vi "HSOpMuxNoRef.vi"() -> ()   [LabVIEW 2013]
uses:
  Multiplexer_Opmux.lvclass
  OverallRoutines/HS3OverallRoutines.lvlib
panel:
  out "tmr":u32 caption="Elapsed for acq"
  in  "Run":bool
  out "Ch8":dbl[](graph)
  out "Ch7":dbl[](graph)
  out "Ch6":dbl[](graph)
  out "Ch5":dbl[](graph)
  out "Ch4":dbl[](graph)
  out "Ch3":dbl[](graph)
  out "Ch2":dbl[](graph)
  out "Ch1":dbl[](graph)
  in  "Scan":bool
  in  "Set":bool
  in  "Length":dbl=1.0 caption="Length (us)" min=0.1 max=6.3 step=0.1
  in  "Voltage":dbl min=0.0 max=1023.0 step=1.0
  in  "Into":u16[](array[numeric])
  in  "Forward":u16[](array[numeric])
  in  "Signal Frequency":u32(ring)=10000000 items=["5Mhz"=5000000, "10Mhz"=10000000, "25Mhz"=25000000]
  in  "Shutdown":bool
  out "Acq":bool caption="Acquiring"
  out "SampleFrequency":dbl format="%#_8g"
  out "ChArray":dbl[](array[numeric])
  out "Serial":i32
  out "DllPath":path
  out "HandyScope":bool
  out "Multiplexer":bool
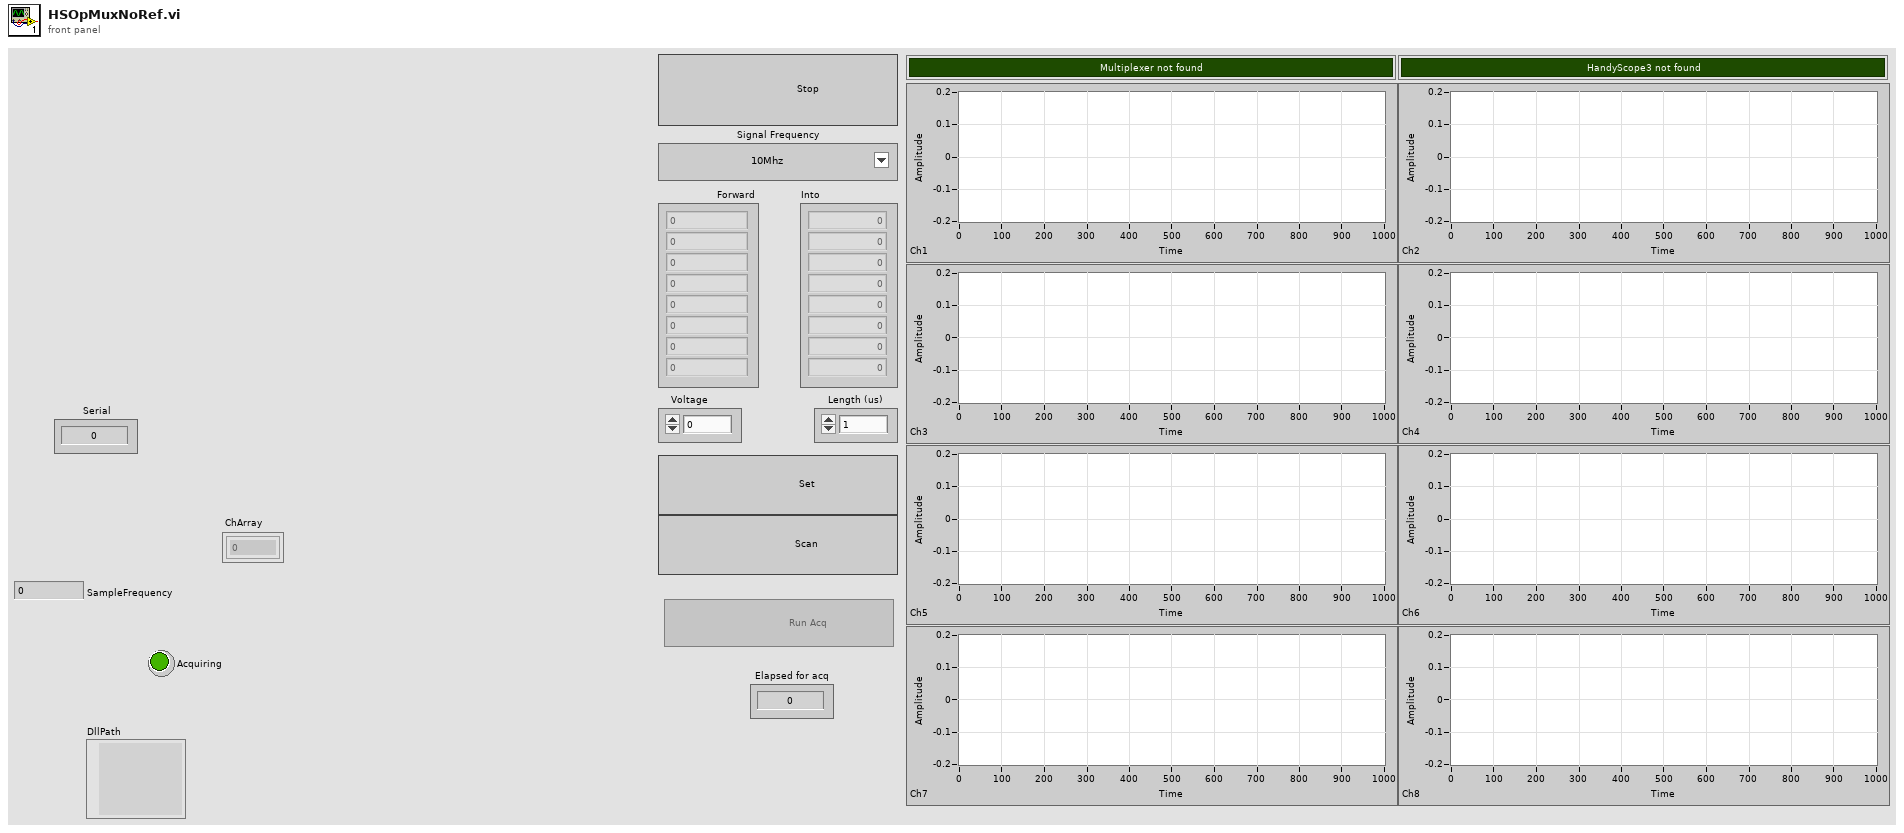
[diagram p1: front panel]
types:
  T1 = cluster{"trgSource":u16, "trgMode":u16, "trgLevel":dbl}
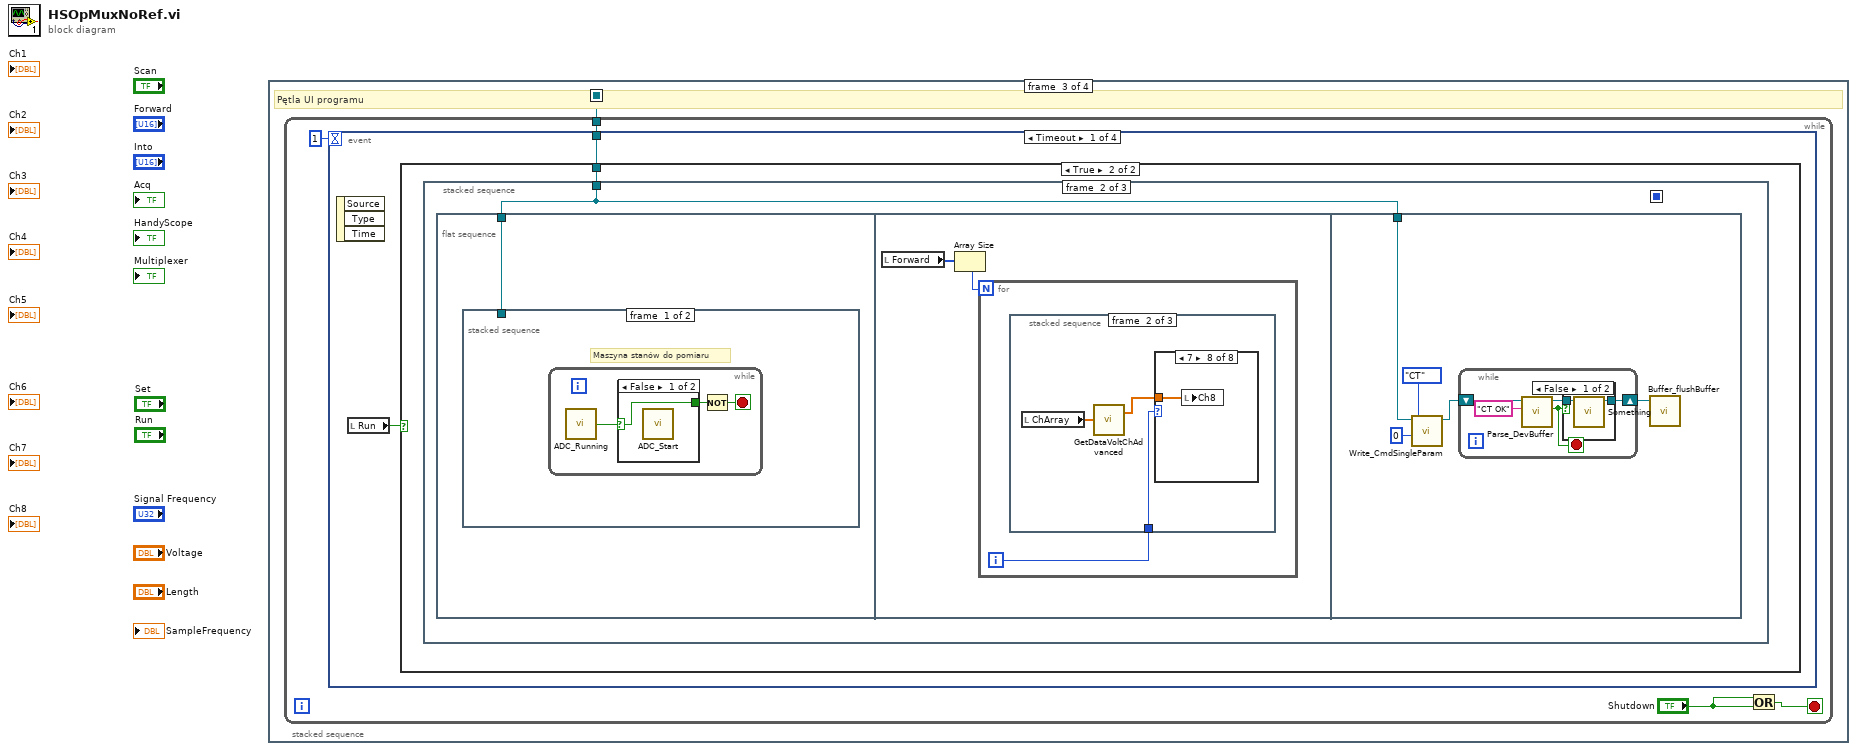
[diagram p0: block diagram]
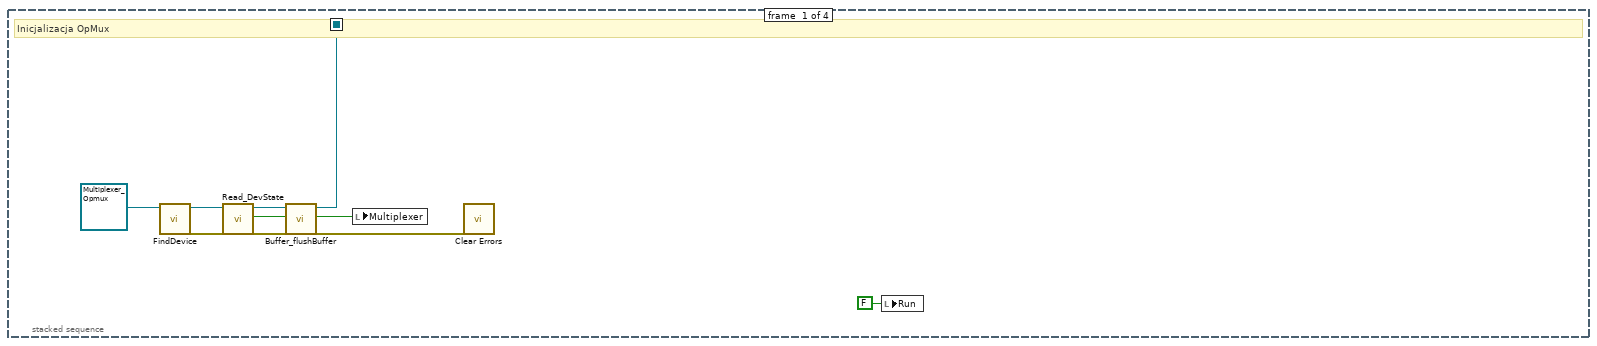
[diagram p2: hidden frame]
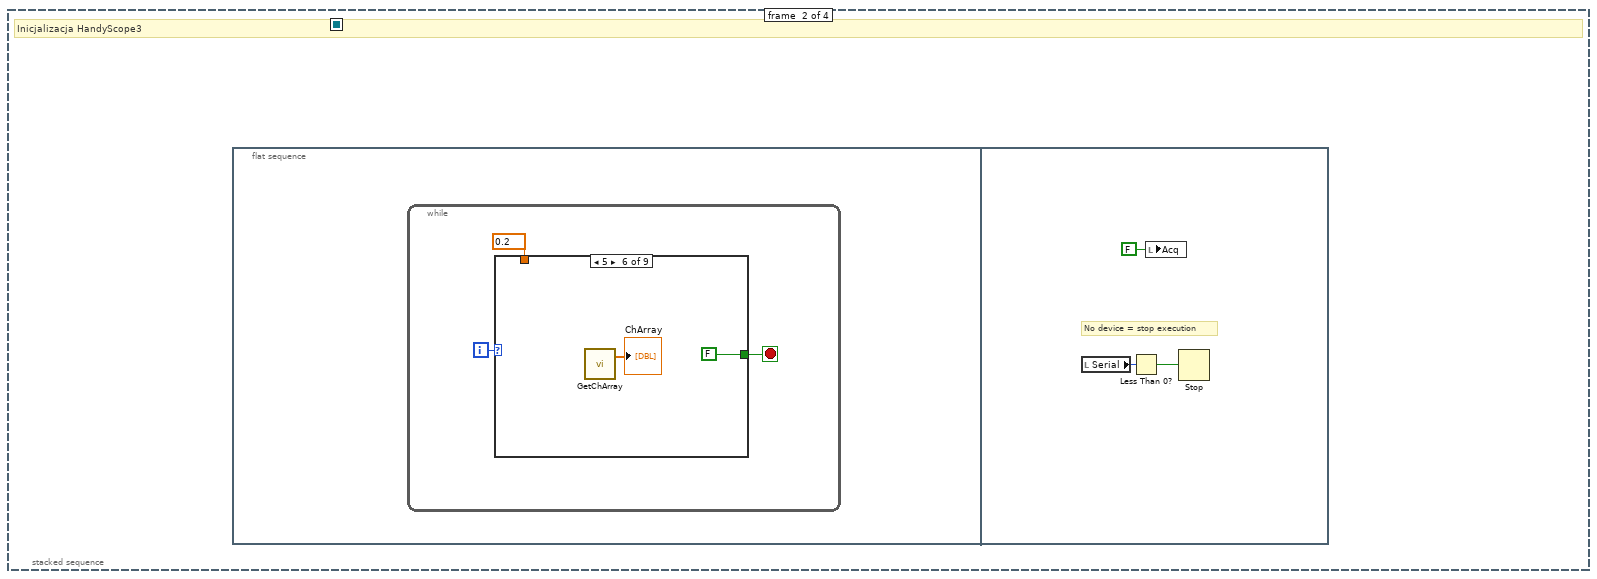
[diagram p3: hidden frame]
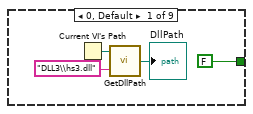
[diagram p4: hidden frame]
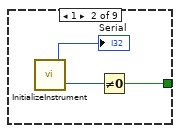
[diagram p5: hidden frame]
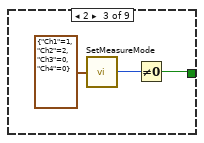
[diagram p6: hidden frame]
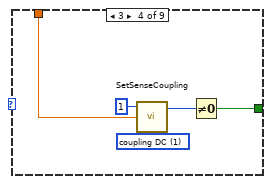
[diagram p7: hidden frame]
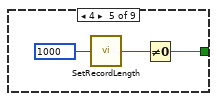
[diagram p8: hidden frame]
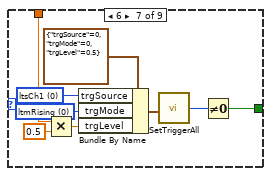
[diagram p9: hidden frame]
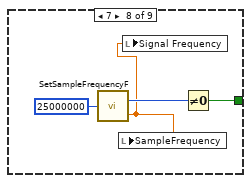
[diagram p10: hidden frame]
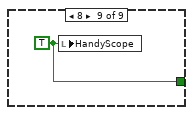
[diagram p11: hidden frame]
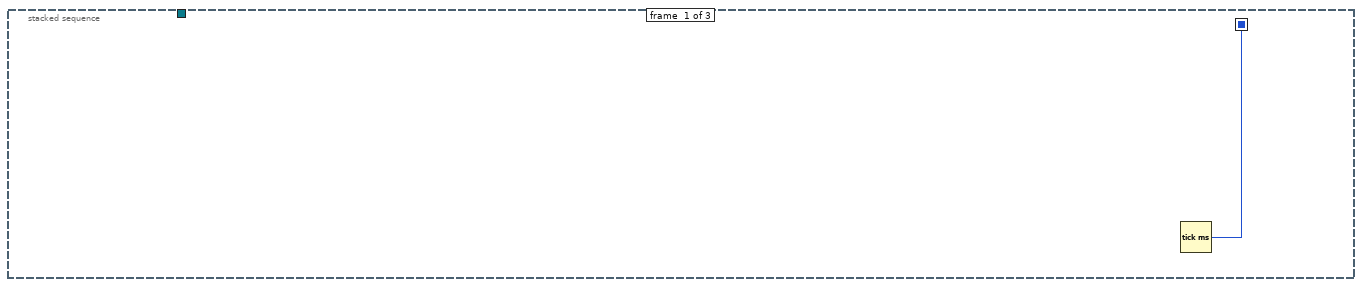
[diagram p13: hidden frame]
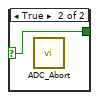
[diagram p14: hidden frame]
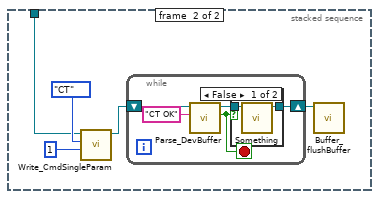
[diagram p15: hidden frame]
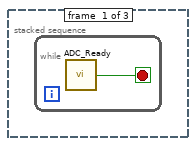
[diagram p17: hidden frame]
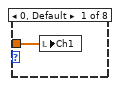
[diagram p18: hidden frame]
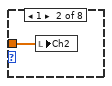
[diagram p19: hidden frame]
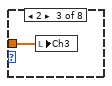
[diagram p20: hidden frame]
diagram:
  n1 = stacked-sequence {
    seq-local: [w1 _ _ _] -> [_ _ w50 _]
    frame #0 {
      # "Inicjalizacja OpMux"
      n2 = call-dynamic "FindDevice.vi"("Multiplexer_Opmux in"=refnum<class "Multiplexer_Opmux.lvclass"> refnum) -> ("error out"=w6:errorcluster, "Multiplexer_Opmux out"=w8:refnum<class "Multiplexer_Opmux.lvclass">)  [unwired: 8 in, 1 out]
      n3 = call-dynamic "Read_DevState.vi"("error in (no error)"=w6, "Multiplexer_Opmux in"=w8) -> ("error out"=w3:errorcluster, "DevState"=w7:bool, "Multiplexer_Opmux out"=w4:refnum<class "Multiplexer_Opmux.lvclass">)  [unwired: 7 in]
      n4 = call-dynamic "Buffer_flushBuffer.vi"("error in (no error)"=w3, "Multiplexer_Opmux in"=w4) -> ("error out"=w2:errorcluster, "Multiplexer_Opmux out"=w1:refnum<class "Multiplexer_Opmux.lvclass">)  [unwired: 8 in]
      n5 = local write "Multiplexer"(w7) -> ()
      n6 = call <vilib>:"Clear Errors.vi"("error in (no error)"=w2) -> ()  [unwired: 6 in, 1 out]
      n7 = local write "Run"(FALSE ("Run")) -> ()
    }
    frame #1 {
      # "Inicjalizacja HandyScope3"
      n8 = flat-sequence {
        frame #0 {
          n9 = while {
            i -> [w12]
            stop <- w11 stop-if-true
            w10 = 0.2 items=["0,2"=0.2, "0,8"=0.8, "2"=2.0, "4"=4.0, "20"=20.0, "40"=40.0, "80"=80.0] ("chSense")
            n10 = case shown="5" w12 {
              tunnel: [FALSE w17 w21 w24 w29 FALSE w40 w45 w46] -> w11
              tunnel: w10 -> [_ _ _ w23 _ _ w36 _ _]
              frame 0, Default {
                n11 = Current VI's Path() -> (path=w14:path)
                n12 = call "GetDllPath.vi"("DllName"="DLL3\\hs3.dll", "path"=w14) -> ("DllPath"=→"DllPath":path)
              }
              frame 1 {
                n13 = call "InitializeInstrument.vi"() -> ("ErrorCode"=w18:i16, "Serial"=→"Serial":i32)
                n14 = Not Equal To 0?(x=w18) -> (x != 0?=w17:bool)
              }
              frame 2 {
                n15 = call "SetMeasureMode.vi"("oModeStack"=cluster{"Ch1":u8, "Ch2":u8, "Ch3":u8, "Ch4":u8} {"Ch1"=1, "Ch2"=2, "Ch3"=0, "Ch4"=0}) -> ("ErrorCode"=w20:i16)
                n16 = Not Equal To 0?(x=w20) -> (x != 0?=w21:bool)
              }
              frame 3 {
                w27 = 1 items=["coupling AC", "coupling DC"] ("chCoupling")
                n17 = call "SetSenseCoupling.vi"("chCoupling"=w27, "chSense"=w23, "chSet"=1) -> ("ErrorCode"=w25:i16)  [unwired: 1 out]
                n18 = Not Equal To 0?(x=w25) -> (x != 0?=w24:bool)
              }
              frame 4 {
                w30 = u32 1000 items=["100"=100, "250"=250, "500"=500, "1000"=1000, "2500"=2500, "5000"=5000, "10000"=10000, "25000"=25000, "50000"=50000, "100000"=100000, "131000"=131000] ("RecordLength")
                n19 = call "SetRecordLength.vi"("RecordLength"=w30) -> ("ErrorCode"=w28:i16)
                n20 = Not Equal To 0?(x=w28) -> (x != 0?=w29:bool)
              }
              frame 5 {
                n21 = call "GetChArray.vi"() -> ("ChArray"=→"ChArray":dbl[])  [unwired: 1 out]
              }
              frame 6 {
                w33 = u16 0 items=["ltmRising", "ltmFalling", "ltmInWindow", "ltmOutWindow", "ltmTVLine", "ltmTVFieldOdd", "ltmTVFieldEven"] ("trgMode")
                w34 = u16 0 items=["ltsCh1"=0, "ltsCh2"=1, "ltsExternal"=4, "ltsAnalogExt"=5, "ltsAnd"=6, "ltsOr"=7, "ltsXor"=8, "ltsNoTrig"=9, "notUsed"=10, "ltsPxiExt"=11, "ltsGenStart"=12, "ltsGenStop"=13, "ltsGenNew"=14] ("trgSource")
                n22 = Multiply(x=w36, y=0.5) -> (x*y=w37:dbl)
                n23 = Bundle By Name(cluster=T1 {"trgSource"=0, "trgMode"=0, "trgLevel"=0.5} ("TriggerSettings"), "trgSource"=w34, "trgMode"=w33, "trgLevel"=w37) -> (w38:T1)
                n24 = call "SetTriggerAll.vi"("TriggerSettings"=w38) -> ("ErrorCode"=w41:i32)
                n25 = Not Equal To 0?(x=w41) -> (x != 0?=w40:bool)
              }
              frame 7 {
                n26 = call "SetSampleFrequencyF.vi"("Numeric Control"=u32 25000000) -> ("ErrorCode"=w44:i16, "oFreq_Set"=w43:dbl)
                n27 = local write "SampleFrequency"(w43) -> ()
                n28 = local write "Signal Frequency"(w43) -> ()
                n29 = Not Equal To 0?(x=w44) -> (x != 0?=w45:bool)
              }
              frame 8 {
                w46 = TRUE ("HandyScope")
                n30 = local write "HandyScope"(w46) -> ()
              }
            }
          }
        }
        frame #1 {
          # "No device = stop execution"
          n31 = local read "Serial"() -> (w49:i32)
          n32 = Less Than 0?(x=w49) -> (x < 0?=w48:bool)
          n33 = local write "Acq"(FALSE ("Acq")) -> ()
          n34 = Stop(stop? (T)=w48) -> ()
        }
      }
    }
    frame #2 {
      # "Pętla UI programu"
      n35 = while {
        tunnel: w50 -> [w51]
        stop <- w53 stop-if-true
        n36 = event shown="[0] Timeout" {
          selector: _ -> [_ _ _ _]
          dyn-events: _ -> [_ _ _ _]
          timeout: 1 -> [_ _ _ _]
          tunnel: w51 -> [w56 _ w111 _]
          event Timeout {
            n37 = event-data() -> ()  [unwired: 1 in, 3 out]
            n38 = local read "Run"() -> (w55:bool)
            n39 = case shown="True" w55 {
              tunnel: w56 -> [_ w57]
              frame False {
              }
              frame True {
                n40 = stacked-sequence {
                  seq-local: [w58 _ _] -> [_ _ w108]
                  tunnel: w57 -> [_ w59 _]
                  frame #0 {
                    n41 = Tick Count (ms)() -> (millisecond timer value=w58:u32)
                  }
                  frame #1 {
                    n42 = flat-sequence {
                      tunnel: w59 -> [w60]
                      tunnel: w59 -> [w96]
                      frame #0 {
                        n43 = stacked-sequence {
                          tunnel: w60 -> [_ w66]
                          frame #0 {
                            # "Maszyna stanów do pomiaru"
                            n44 = while {
                              stop <- w62 stop-if-true
                              n45 = call "ADC_Running.vi"() -> ("Measuring"=w63:bool)
                              n46 = case shown="False" w63 {
                                selector: w63 -> [w64 w65]
                                tunnel: [w64 w65] -> w61
                                frame False {
                                n47 = call "ADC_Start.vi"() -> ()  [unwired: 1 out]
                                }
                                frame True {
                                n48 = call "ADC_Abort.vi"() -> ()  [unwired: 1 out]
                                }
                              }
                              n49 = Not(x=w61) -> (.not. x?=w62:bool)
                            }
                          }
                          frame #1 {
                            n50 = call-dynamic "Write_CmdSingleParam.vi"("Param"=1, "Command"=enum16{"SA", "GT", "SI", "SL", "ST", "CT"}."CT", "Multiplexer_Opmux in"=w66) -> ("Multiplexer_Opmux out"=w68:refnum<class "Multiplexer_Opmux.lvclass">)  [unwired: 7 in, 1 out]
                            n51 = while {
                              shift-right: [w72] -> w67
                              shift-left: w68 -> [w71]
                              stop <- w74 stop-if-true
                              n52 = call-dynamic "Parse_DevBuffer.vi"("searchFor"="CT OK", "Multiplexer_Opmux in"=w71) -> ("Found"=w74:bool, "Multiplexer_Opmux out"=w75:refnum<class "Multiplexer_Opmux.lvclass">)  [unwired: 7 in, 1 out]
                              n53 = case shown="False" w74 {
                                tunnel: w75 -> [w77 w78]
                                tunnel: [w76 w78] -> w72
                                frame False {
                                n54 = call-dynamic "Something.vi"("Multiplexer_Opmux in"=w77) -> ("Multiplexer_Opmux out"=w76:refnum<class "Multiplexer_Opmux.lvclass">)  [unwired: 9 in, 1 out]
                                }
                                frame True {
                                }
                              }
                            }
                            n55 = call-dynamic "Buffer_flushBuffer.vi"("Multiplexer_Opmux in"=w67) -> ()  [unwired: 9 in, 2 out]
                          }
                        }
                      }
                      frame #1 {
                        n56 = local read "Forward"() -> (w80:u16[])
                        n57 = Array Size(array=w80) -> (size(s)=w79:i32)
                        n58 = for {
                          N: w79 -> [_]
                          i -> [w81]
                          n59 = stacked-sequence {
                            tunnel: w81 -> [_ w85 _]
                            frame #0 {
                              n60 = while {
                                stop <- w82 stop-if-true
                                n61 = call "ADC_Ready.vi"() -> ("Ready"=w82:bool)
                              }
                            }
                            frame #1 {
                              n62 = local read "ChArray"() -> (w83:dbl[])
                              n63 = call "GetDataVoltChAdvanced.vi"("chData"=w83) -> ("chOutData"=w84:dbl[])  [unwired: 1 out]
                              n64 = case shown="7" w85 {
                                tunnel: w84 -> [w86 w87 w88 w89 w90 w91 w92 w93]
                                frame 0, Default {
                                n65 = local write "Ch1"(w86) -> ()
                                }
                                frame 1 {
                                n66 = local write "Ch2"(w87) -> ()
                                }
                                frame 2 {
                                n67 = local write "Ch3"(w88) -> ()
                                }
                                frame 3 {
                                n68 = local write "Ch4"(w89) -> ()
                                }
                                frame 4 {
                                n69 = local write "Ch5"(w90) -> ()
                                }
                                frame 5 {
                                n70 = local write "Ch6"(w91) -> ()
                                }
                                frame 6 {
                                n71 = local write "Ch7"(w92) -> ()
                                }
                                frame 7 {
                                n72 = local write "Ch8"(w93) -> ()
                                }
                              }
                            }
                            frame #2 {
                              n73 = call "ADC_Start.vi"() -> ()  [unwired: 1 out]
                            }
                          }
                        }
                      }
                      frame #2 {
                        n74 = call-dynamic "Write_CmdSingleParam.vi"("Param"=0, "Command"=enum16{"SA", "GT", "SI", "SL", "ST", "CT"}."CT", "Multiplexer_Opmux in"=w96) -> ("Multiplexer_Opmux out"=w95:refnum<class "Multiplexer_Opmux.lvclass">)  [unwired: 7 in, 1 out]
                        n75 = while {
                          shift-right: [w100] -> w94
                          shift-left: w95 -> [w99]
                          stop <- w102 stop-if-true
                          n76 = call-dynamic "Parse_DevBuffer.vi"("searchFor"="CT OK", "Multiplexer_Opmux in"=w99) -> ("Found"=w102:bool, "Multiplexer_Opmux out"=w103:refnum<class "Multiplexer_Opmux.lvclass">)  [unwired: 7 in, 1 out]
                          n77 = case shown="False" w102 {
                            tunnel: w103 -> [w105 w106]
                            tunnel: [w104 w106] -> w100
                            frame False {
                              n78 = call-dynamic "Something.vi"("Multiplexer_Opmux in"=w105) -> ("Multiplexer_Opmux out"=w104:refnum<class "Multiplexer_Opmux.lvclass">)  [unwired: 9 in, 1 out]
                            }
                            frame True {
                            }
                          }
                        }
                        n79 = call-dynamic "Buffer_flushBuffer.vi"("Multiplexer_Opmux in"=w94) -> ()  [unwired: 9 in, 2 out]
                      }
                    }
                  }
                  frame #2 {
                    n80 = Tick Count (ms)() -> (millisecond timer value=w109:u32)
                    n81 = Subtract(x=w109, y=w108) -> (x-y=→"tmr":u32)
                  }
                }
              }
            }
          }
          event "Scan": Value Change {
            n82 = event-data() -> ()  [unwired: 1 in, 6 out]
          }
          event "Set": Value Change {
            n83 = event-data() -> ()  [unwired: 1 in, 6 out]
            n84 = local write "Set"(FALSE ("Set")) -> ()
            n85 = stacked-sequence {
              tunnel: w111 -> [w114 _ w116 _ w121 _ w127 _ w131 _ w133]
              frame #0 {
                n86 = call-dynamic "Write_CmdSingleParam.vi"("Param"=0, "Command"=enum16{"SA", "GT", "SI", "SL", "ST", "CT"}."CT", "Multiplexer_Opmux in"=w114) -> ()  [unwired: 7 in, 2 out]
              }
              frame #1 {
                n87 = Wait (ms)(milliseconds to wait=u32 50) -> ()  [unwired: 1 out]
              }
              frame #2 {
                n88 = local read "Forward"() -> (w119:u16[])
                n89 = local read "Into"() -> (w118:u16[])
                n90 = call-dynamic "Write_CmdMultipleParam.vi"("Command"=enum16{"ST"}."ST", "Table2"=w118, "Table1"=w119, "Multiplexer_Opmux in"=w116) -> ()  [unwired: 6 in, 2 out]
              }
              frame #3 {
                n91 = Wait (ms)(milliseconds to wait=u32 50) -> ()  [unwired: 1 out]
              }
              frame #4 {
                n92 = local read "Length"() -> (w123:dbl)
                n93 = Multiply(x=w123, y=10.0) -> (x*y=w124:dbl)
                n94 = call-dynamic "Write_CmdSingleParam.vi"("Param"=w124, "Command"=enum16{"SA", "GT", "SI", "SL", "ST", "CT"}."SL", "Multiplexer_Opmux in"=w121) -> ()  [unwired: 7 in, 2 out]
              }
              frame #5 {
                n95 = Wait (ms)(milliseconds to wait=u32 50) -> ()  [unwired: 1 out]
              }
              frame #6 {
                n96 = local read "Voltage"() -> (w129:dbl)
                n97 = call-dynamic "Write_CmdSingleParam.vi"("Param"=w129, "Command"=enum16{"SA", "GT", "SI", "SL", "ST", "CT"}."SI", "Multiplexer_Opmux in"=w127) -> ()  [unwired: 7 in, 2 out]
              }
              frame #7 {
                n98 = Wait (ms)(milliseconds to wait=u32 50) -> ()  [unwired: 1 out]
              }
              frame #8 {
                n99 = call-dynamic "Buffer_flushBuffer.vi"("Multiplexer_Opmux in"=w131) -> ()  [unwired: 9 in, 2 out]
              }
              frame #9 {
                n100 = Wait (ms)(milliseconds to wait=u32 25) -> ()  [unwired: 1 out]
              }
              frame #10 {
                n101 = local write "Run"(TRUE ("Run")) -> ()
                n102 = call-dynamic "Write_CmdSingleParam.vi"("Param"=1, "Command"=enum16{"SA", "GT", "SI", "SL", "ST", "CT"}."CT", "Multiplexer_Opmux in"=w133) -> ()  [unwired: 7 in, 2 out]
                n103 = call "ADC_Abort.vi"() -> ()  [unwired: 1 out]
              }
            }
          }
          event "Signal Frequency": Value Change {
            n104 = event-data() -> ("NewVal"=w137:u32)  [unwired: 1 in, 5 out]
            n105 = stacked-sequence {
              tunnel: w137 -> [w141 _]
              frame #0 {
                n106 = call "SetSampleFrequencyF.vi"("Numeric Control"=w141) -> ("ErrorCode"=w140:i16, "oFreq_Set"=w139:dbl)
                n107 = case shown="True" TRUE {
                  tunnel: w139 -> [_ w145]
                  frame False {
                  }
                  frame True {
                    # "Do 100us sygnał zmieniamy automatycznie"
                    n108 = Multiply(x=w145, y=4e-05) -> (x*y=w143:dbl)
                    n109 = To Unsigned Long Integer(number=w143) -> (unsigned 32bit integer=w144:u32)
                    n110 = call "SetRecordLength.vi"("RecordLength"=w144) -> ()  [unwired: 1 out]
                  }
                }
                n111 = local write "SampleFrequency"(w139) -> ()
                n112 = call "Error Converter (ErrCode or Status).vi"("error code"=w140) -> ()  [unwired: 10 in, 1 out]
              }
              frame #1 {
              }
            }
          }
        }
        n113 = Or(x="Shutdown", y="Shutdown") -> (x .or. y?=w53:bool)
      }
    }
    frame #3 {
      # "Rozłączenie urządzeń po zakończeniu działania programu"
    }
  }
